vi "downloadExample.vi"() -> ()   [LabVIEW 2016, in "GDrive.lvlib"]
doc: "Example of how to download a file from Google Drive to the local machine (location determined by the control Desired file path)"
uses:
  VIs/GDrive.lvlib
panel:
  in  "File Name":string
  in  "Local Path":path
  in  "Path to Secret Client JSON":path
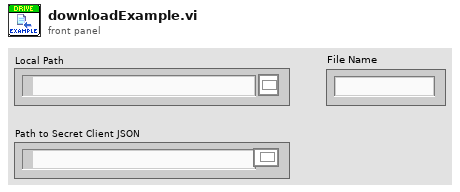
[diagram p1: front panel]
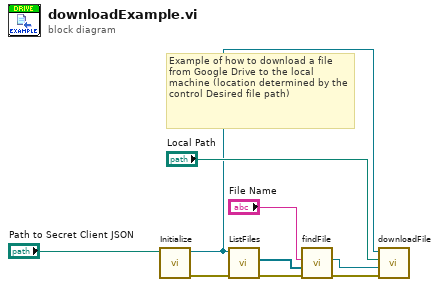
[diagram p0: block diagram]
diagram:
  # "Example of how to download a file from Google Drive to the local machine (location determined by the control Desired file path)"
  n1 = call "Initialize.vi"("Path to Secret Client JSON"="Path to Secret Client JSON") -> ("error out"=w8:errorcluster, "Google Drive Service Ref"=w3:refnum<k24>)  [unwired: 9 in]
  n2 = call "ListFiles.vi"("error in (no error)"=w8, "Google Drive Service Ref In"=w3) -> ("error out"=w7:errorcluster, "Files"=w1:refnum<k24>[])  [unwired: 7 in, 1 out]
  n3 = call "findFile.vi"("Error In"=w7, "Files"=w1, "File Name"="File Name") -> ("error out"=w5:errorcluster, "File Reference"=w2:refnum<k24>)  [unwired: 7 in]
  n4 = call "downloadFile.vi"("error in (no error)"=w5, "File Reference"=w2, "Local Path"="Local Path", "Google Drive Service Ref"=w3) -> ()  [unwired: 5 in, 1 out]
